vi "(生長曲線)cos.vi"(11 "目標in":T1={"起始"=0.0, "終點"=200.0, "max speed(估算)"=80.0, "dt"=10.0}) -> (1 "次數":i32, 2 "距離曲線(cm)":dbl[](array[numeric]), 3 "speed曲線(cm/s)":dbl[](array[numeric]))   [LabVIEW 2015]
panel:
  out "V_T":cluster{i32[], dbl[]}(graph)
  out "dt":dbl
  in  "x array":dbl[](array[numeric])
  out "終點":dbl format="%#_13g"
  out "起始":dbl format="%#_13g"
  out "cosine x，y":dbl[][](array[numeric])
  out "X_T":cluster{i32[], dbl[]}(graph)
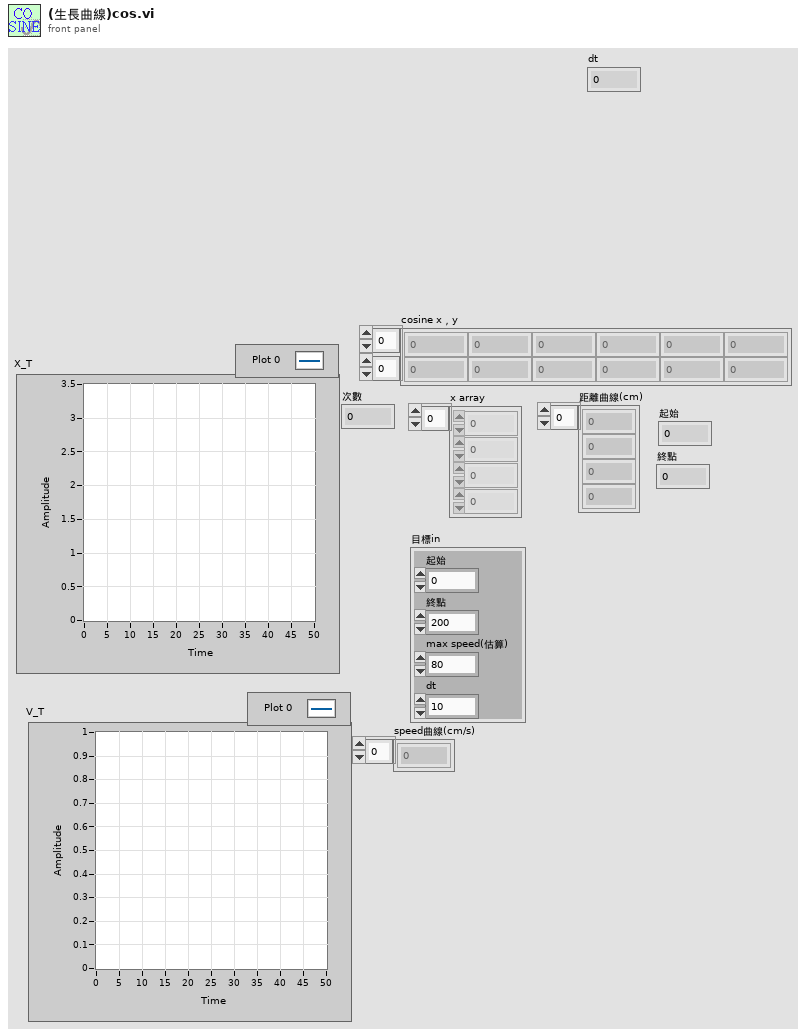
[diagram p1: front panel]
types:
  T1 = cluster{"起始":dbl, "終點":dbl, "max speed(估算)":dbl, "dt":dbl}
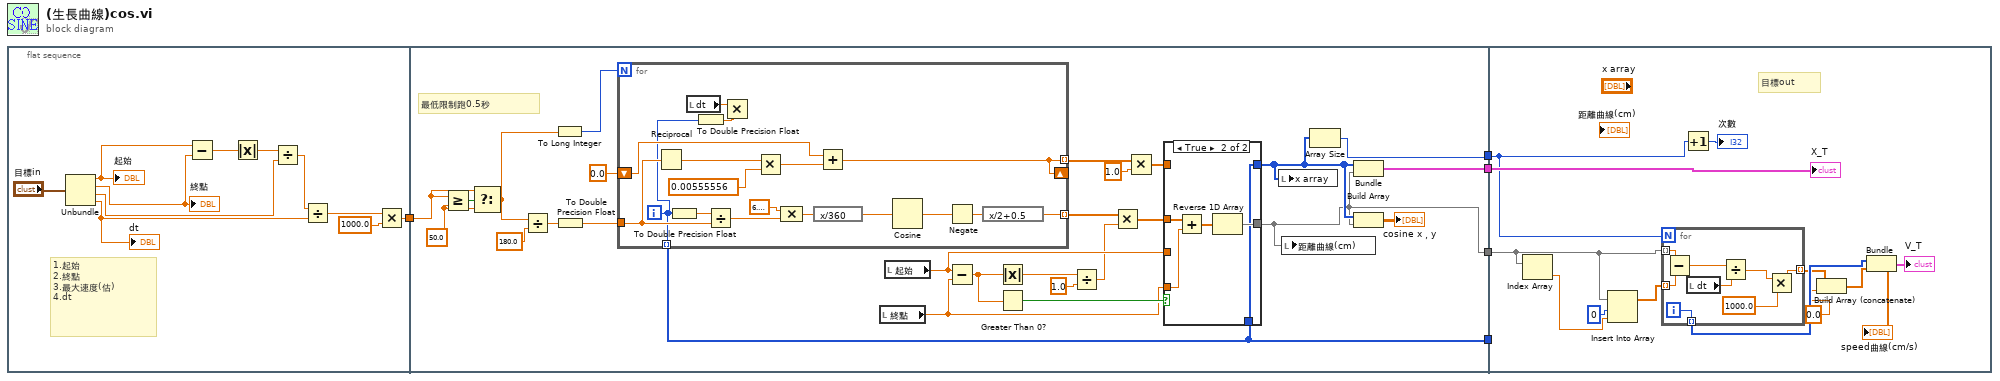
[diagram p0: block diagram]
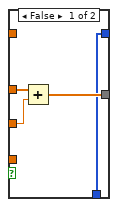
[diagram p2: hidden frame]
diagram:
  n1 = flat-sequence {
    tunnel: [w10] -> w5
    tunnel: w5 -> [w19]
    tunnel: [w26] -> w4
    tunnel: [w25] -> w3
    tunnel: [w24] -> w2
    tunnel: [w21] -> w1
    tunnel: w4 -> [w77]
    tunnel: w3 -> [w81]
    tunnel: w2 -> [_]
    tunnel: w1 -> [w71]
    frame #0 {
      # "1.起始\n2.終點\n3.最大速度(估)\n4.dt"
      n2 = Unbundle("目標in") -> ("起始"=w9:dbl, "終點"=w8:dbl, "max speed(估算)"=w7:dbl, "dt"=w6:dbl)
      "終點" <- w8
      "起始" <- w9
      "dt" <- w6
      n3 = Subtract(x=w9, y=w8) -> (x-y=w15:dbl)
      n4 = Absolute Value(x=w15) -> (abs(x)=w14:dbl)
      n5 = Divide(x=w14, y=w7) -> (x/y=w13:dbl)
      n6 = Divide(x=w13, y=w6) -> (x/y=w12:dbl)
      n7 = Multiply(x=w12, y=1000.0) -> (x*y=w10:dbl)
    }
    frame #1 {
      w18 = 50.0 ("y")
      # "最低限制跑0.5秒"
      n8 = Greater Or Equal?(x=w19, y=w18) -> (x >= y?=w20:bool)
      n9 = Select(t=w19, s=w20, f=w18) -> (s? t:f=w17:dbl)
      n10 = Divide(x=w17, y=180.0) -> (x/y=w28:dbl)
      n11 = To Long Integer(number=w17) -> (32bit integer=w31:i32)
      n12 = To Double Precision Float(number=w28) -> (double precision float=w30:dbl)
      n13 = for {
        N: w31 -> [_]
        tunnel: [w58] -> w23 mode=indexing
        shift-right: [w60] -> _
        shift-left: 0.0 -> [w67]
        tunnel: [w60] -> w37 mode=indexing
        tunnel: w30 -> [w56]
        tunnel: [w53] -> w24 mode=indexing
        i -> [w53]
        n14 = Reciprocal(x=w56) -> (1/x=w57:dbl)
        n15 = To Double Precision Float(number=w53) -> (double precision float=w61:dbl)
        n16 = local read "dt"() -> (w55:dbl)
        n17 = To Double Precision Float(number=w53) -> (double precision float=w54:dbl)
        n18 = Divide(x=w61, y=w56) -> (x/y=w62:dbl)
        n19 = Multiply(x=w55, y=w54) -> ()  [unwired: 1 out]
        n20 = Multiply(x=w57, y=0.00555556) -> (x*y=w64:dbl)
        n21 = Compound Arithmetic op=MULTIPLY(6.283185307179586, w62) -> (w68:dbl)
        n22 = expression code="x/360"(w68) -> (w66:dbl)
        n23 = Add(x=w67, y=w64) -> (x+y=w60:dbl)
        n24 = Cosine(x=w66) -> (cos(x)=w65:dbl)
        n25 = Negate(x=w65) -> (-x=w59:dbl)
        n26 = expression code="x/2+0.5"(w59) -> (w58:dbl)
      }
      n27 = local read "終點"() -> (w34:dbl)
      n28 = local read "起始"() -> (w35:dbl)
      n29 = Subtract(x=w35, y=w34) -> (x-y=w40:dbl)
      n30 = Absolute Value(x=w40) -> (abs(x)=w39:dbl)
      n31 = Greater Than 0?(x=w40) -> (x > 0?=w41:bool)
      n32 = Divide(x=w39, y=1.0) -> (x/y=w32:dbl)
      n33 = Multiply(x=w23, y=w32) -> (x*y=w22:dbl[])
      n34 = Multiply(x=w37, y=1.0) -> (x*y=w36:dbl[])
      n35 = case shown="True" w41 {
        tunnel: w22 -> [w45 w49]
        tunnel: [w46 w50] -> w21
        tunnel: w36 -> [_ _]
        tunnel: w35 -> [w47 _]
        tunnel: [w44 w48] -> w27
        tunnel: w34 -> [_ w52]
        tunnel: w24 -> [w44 w48]
        frame False {
          n36 = Add(x=w45, y=w47) -> (x+y=w46:dbl[])
        }
        frame True {
          n37 = Add(x=w49, y=w52) -> (x+y=w51:dbl[])
          n38 = Reverse 1D Array(array=w51) -> (reversed array=w50:dbl[])
        }
      }
      n39 = local write "x array"(w27) -> ()
      n40 = local write "距離曲線(cm)"(w21) -> ()
      n41 = Array Size(array=w27) -> (size(s)=w26:i32)
      n42 = Bundle(w27, w21) -> (w25:cluster{i32[], dbl[]})  [unwired: 1 in]
      n43 = Build Array(w27, w21) -> (→"cosine x，y":dbl[][])
    }
    frame #2 {
      # "目標out"
      n44 = Index Array(array=w71) -> (element=w70:dbl)  [unwired: 1 in]
      n45 = Insert Into Array(array=w71, index=0, new element=w70) -> (w78:dbl[])
      n46 = for {
        N: w77 -> [_]
        tunnel: w71 -> [w85] mode=indexing
        tunnel: [w87] -> w75 mode=indexing
        tunnel: [w89] -> w79 mode=indexing
        tunnel: w78 -> [w84] mode=indexing
        i -> [w89]
        n47 = Subtract(x=w85, y=w84) -> (x-y=w83:dbl)
        n48 = local read "dt"() -> (w82:dbl)
        n49 = Divide(x=w83, y=w82) -> (x/y=w88:dbl)
        n50 = Multiply(x=w88, y=1000.0) -> (x*y=w87:dbl)
      }
      n51 = Increment(x=w77) -> (x+1=→"次數":i32)
      n52 = Build Array (concatenate)(w75, 0.0) -> (w73:dbl[])
      "speed曲線(cm/s)" <- w73
      n53 = Bundle(w79, w73) -> (→"V_T":cluster{i32[], dbl[]})  [unwired: 1 in]
      "X_T" <- w81
    }
  }
